vi "DT_With_Multiplexer.vi"() -> (0 "error IO":errorcluster)   [LabVIEW 2017]
doc: "This vi will take data with multiple DT boxes for an arbitrary number of channels either differentially or single ended, depending upon how you have wired the boxes up."
uses:
  Globals/Meas_global.vi
panel:
  in  "DT Board num.":u32=1
  out "Waveform Graph":dbl[][](graph)
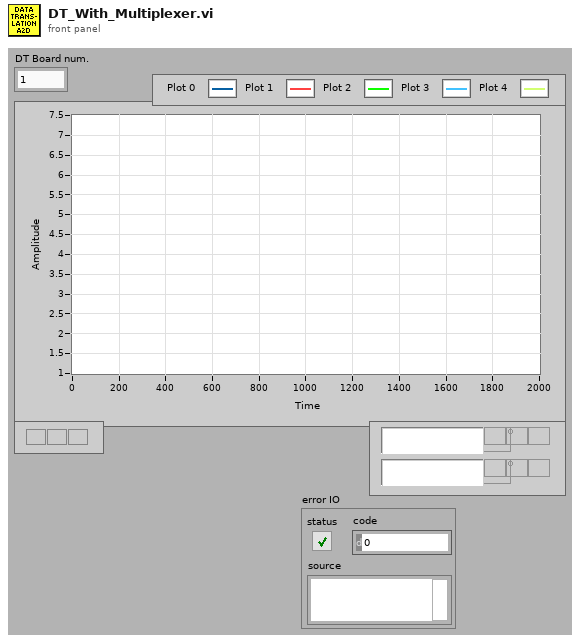
[diagram p1: front panel]
types:
  T1 = typedef "LDA_Setup.ctl" = cluster{"dimensions":enum16{"1D", "2D"}, "Analogue Freq Multiplier":dbl}
  T2 = typedef "Ch_and_Spans.ctl" = cluster{"Sync Delay (ms)":dbl, "Ch No":i16, "Var name":string, "Use Latest Calib":bool}
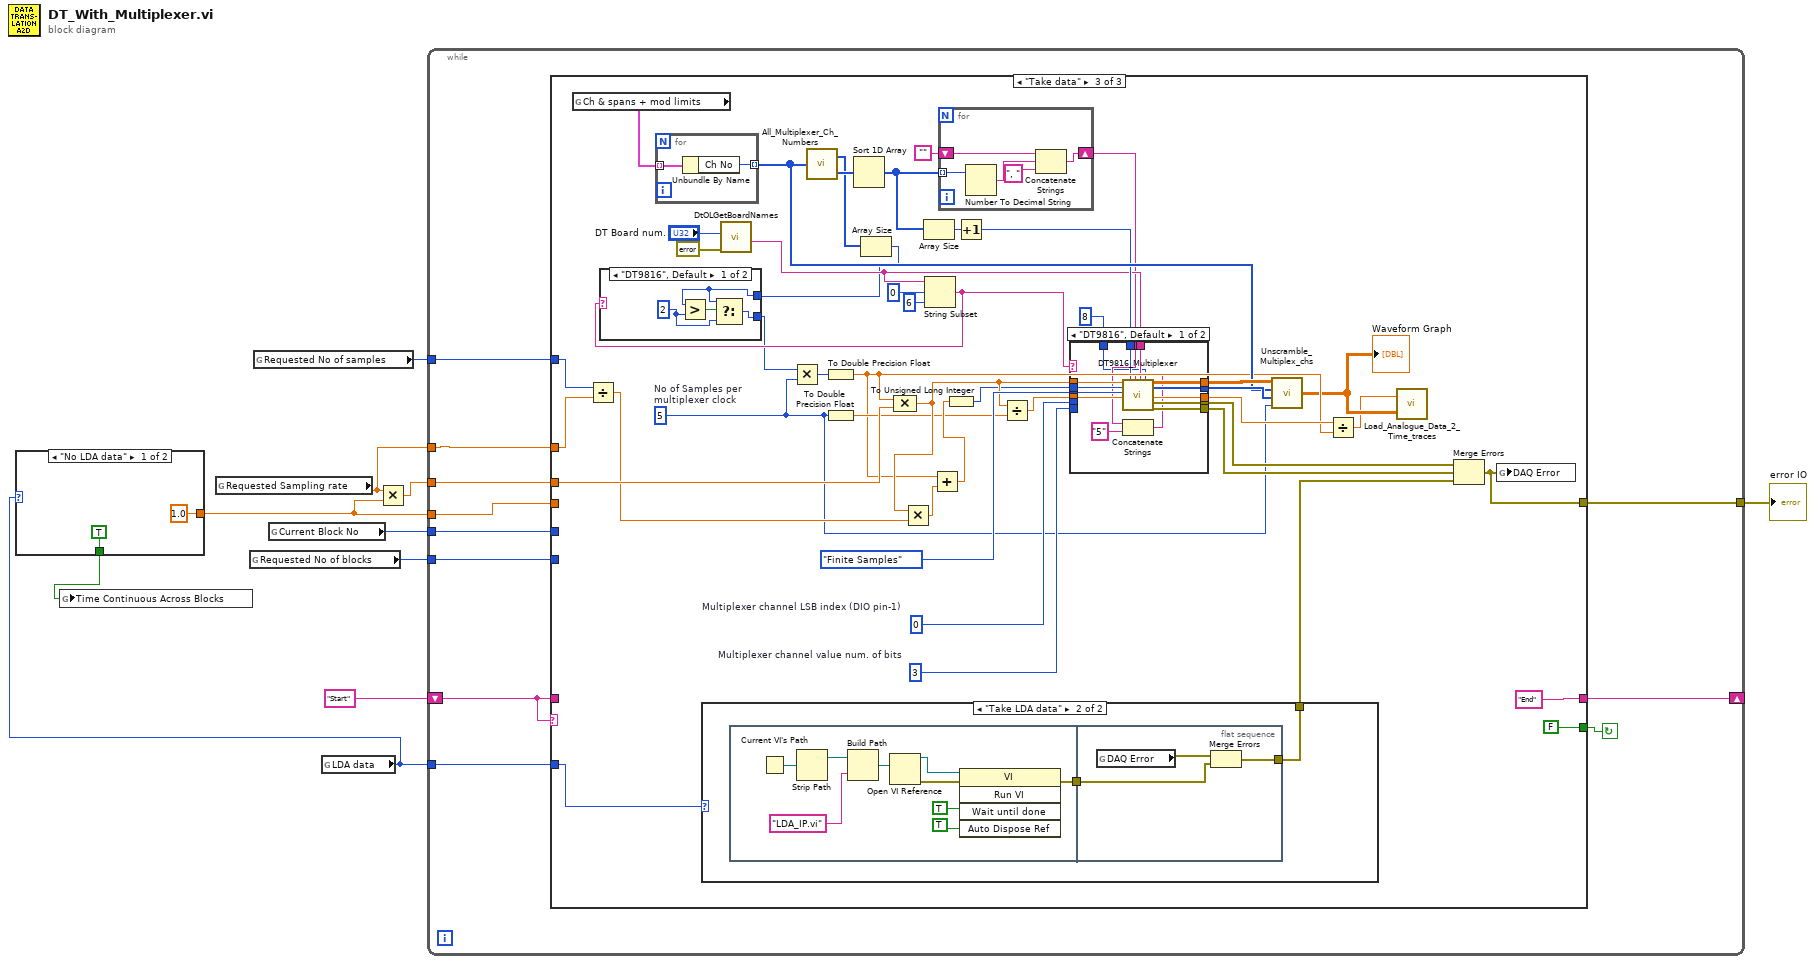
[diagram p0: block diagram]
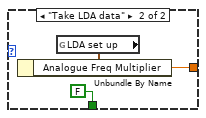
[diagram p2: hidden frame]
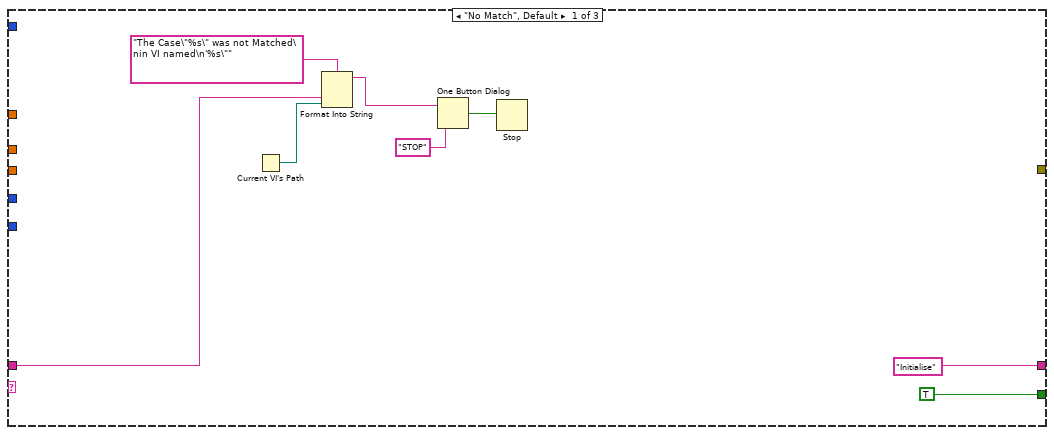
[diagram p3: hidden frame]
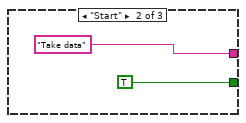
[diagram p4: hidden frame]
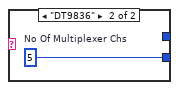
[diagram p5: hidden frame]
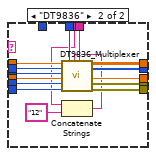
[diagram p6: hidden frame]
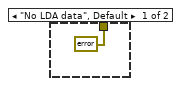
[diagram p7: hidden frame]
diagram:
  n1 = global read "Meas_global.vi" "Requested Sampling rate"() -> (w6:dbl)
  n2 = global read "Meas_global.vi" "Requested No of blocks"() -> (w5:i32)
  n3 = global read "Meas_global.vi" "Requested No of samples"() -> (w9:i32)
  n4 = global read "Meas_global.vi" "Current Block No"() -> (w8:i32)
  n5 = global read "Meas_global.vi" "LDA data"() -> (w3:enum16{"No LDA data", "Take LDA data"})
  n6 = case shown="\"No LDA data\"" w3 {
    tunnel: [1.0 ("Analogue Freq Multiplier") w14] -> w4
    tunnel: [TRUE FALSE] -> w2
    frame "No LDA data" {
    }
    frame "Take LDA data" {
      n7 = global read "Meas_global.vi" "LDA set up"() -> (w15:T1)
      n8 = Unbundle By Name(w15) -> ("Analogue Freq Multiplier"=w14:dbl)
    }
  }
  n9 = global write "Meas_global.vi" "Time Continuous Across Blocks"(w2) -> ()
  n10 = Multiply(x=w6, y=w4) -> (x*y=w7:dbl)
  n11 = while {
    shift-left: "Start" -> [w25]
    shift-right: [w26] -> _
    tunnel: w7 -> [w24]
    tunnel: w9 -> [w23]
    tunnel: w8 -> [w22]
    tunnel: w3 -> [w20]
    tunnel: w4 -> [w19]
    tunnel: w6 -> [w18]
    tunnel: w5 -> [w17]
    tunnel: [w16] -> w1
    stop <- w21 continue-if-true
    n12 = case shown="\"Take data\"" w25 {
      tunnel: ["Initialise" "Take data" "End"] -> w26
      tunnel: w25 -> [w30 _ _]
      tunnel: w24 -> [_ _ w77]
      tunnel: w23 -> [_ _ w76]
      tunnel: w22 -> [_ _ _]
      tunnel: [TRUE TRUE FALSE] -> w21
      tunnel: w20 -> [_ _ w80]
      tunnel: w19 -> [_ _ _]
      tunnel: w18 -> [_ _ w59]
      tunnel: w17 -> [_ _ _]
      tunnel: [_ _ w39] -> w16
      frame "No Match", Default {
        n13 = Current VI's Path() -> (path=w29:path)
        n14 = Format Into String(format string="The Case\"%s\" was not Matched\nin VI named\n'%s\"" ("Format String"), w30, w29) -> (resulting string=w33:string)  [unwired: 2 in, 1 out]
        n15 = One Button Dialog(message=w33, button name ("OK")="STOP") -> (true=w31:bool)
        n16 = Stop(stop? (T)=w31) -> ()
      }
      frame "Start" {
      }
      frame "Take data" {
        w63 = 3  # Multiplexer channel value num. of bits
        w64 = 0  # Multiplexer channel LSB index (DIO pin-1)
        w41 = 5  # No of Samples per multiplexer clock
        n17 = global read "Meas_global.vi" "Ch & spans + mod limits"() -> (w79:T2[])
        n18 = Divide(x=w76, y=w59) -> (x/y=w75:dbl)
        n19 = for {
          tunnel: w79 -> [w125] mode=indexing
          tunnel: [w124] -> w67 mode=indexing
          n20 = Unbundle By Name(w125) -> ("Ch No"=w124:i16)
        }
        n21 = case shown="\"Take LDA data\"" w80 {
          tunnel: [errorcluster {"status"=FALSE, "code"=0, "source"=""} ("error IO") w127] -> w60
          frame "No LDA data", Default {
          }
          frame "Take LDA data" {
            n22 = flat-sequence {
              tunnel: [w129] -> w128
              tunnel: w128 -> [w139]
              tunnel: [w138] -> w127
              frame #0 {
                n23 = Current VI's Path() -> (path=w131:path)
                n24 = Strip Path(path=w131) -> (stripped path=w130:path)  [unwired: 1 out]
                n25 = Build Path(base path=w130, name or relative path="LDA_IP.vi") -> (appended path=w132:path)
                n26 = Open VI Reference(vi path=w132) -> (vi reference=w135:refnum<vi>, error out=w136:errorcluster)  [unwired: 5 in]
                n27 = invoke class="VI" method="Run VI"(reference=w135, error in=w136, "Wait until done"=TRUE ("Wait Until Done"), "Auto Dispose Ref"=TRUE ("Wait until done")) -> (error out=w129:errorcluster)  [unwired: 1 in, 4 out]
              }
              frame #1 {
                n28 = global read "Meas_global.vi" "DAQ Error"() -> (w140:errorcluster)
                n29 = Merge Errors(w140, w139) -> (w138:errorcluster)
              }
            }
          }
        }
        n30 = call <userlib>:"DtOLGetBoardNames.vi"("error in (no error)"=errorcluster {"status"=FALSE, "code"=0, "source"=""}, "Select Board"="DT Board num.") -> ("Board Name"=w49:string)  [unwired: 7 in, 2 out]
        n31 = call "All_Multiplexer_Ch_Numbers.vi"("Channel Numbers"=w67) -> ("Multiplexer Ch No"=w44:i16[], "ADC Ch No"=w58:i16[])
        n32 = To Double Precision Float(number=w41) -> (double precision float=w53:dbl)
        n33 = Sort 1D Array(array=w58) -> (sorted array=w57:i16[])
        n34 = Array Size(array=w44) -> (size(s)=w42:i32)
        n35 = Array Size(array=w57) -> (size(s)=w66:i32)
        n36 = String Subset(string=w49, offset (0)=0, length (rest)=6 ("length (rest)")) -> (substring=w45:string)
        n37 = case shown="\"DT9816\", Default" w45 {
          tunnel: [w83 w87] -> w40
          tunnel: w42 -> [w85 _]
          frame "DT9816", Default {
            w84 = 2 ("y")
            n38 = Greater?(x=w85, y=w84) -> (0:w86:bool)
            n39 = Select(t=w85, s=w86, f=w84) -> (s? t:f=w83:i32)
          }
          frame "DT9836" {
            w87 = 5  # No Of Multiplexer Chs
          }
        }
        n40 = Multiply(x=w40, y=w41) -> (x*y=w52:i32)
        n41 = To Double Precision Float(number=w52) -> (double precision float=w51:dbl)
        n42 = Compound Arithmetic op=MULTIPLY(w51, w77) -> (w71:dbl)
        n43 = Multiply(x=w71, y=w75) -> (x*y=w74:dbl)
        n44 = Add(x=w51, y=w74) -> (x+y=w73:dbl)
        n45 = for {
          tunnel: w57 -> [w123] mode=indexing
          shift-right: [w119] -> w46
          shift-left: "" -> [w120]
          n46 = Number To Decimal String(number=w123) -> (decimal integer string=w122:string)  [unwired: 1 in]
          n47 = Concatenate Strings(w120, w122, ", " ("string")) -> (w119:string)
        }
        n48 = To Unsigned Long Integer(number=w73) -> (unsigned 32bit integer=w50:u32)
        n49 = Increment(x=w66) -> (x+1=w65:i32)
        n50 = Divide(x=w71, y=w53) -> (x/y=w70:dbl)
        n51 = case shown="\"DT9816\", Default" w45 {
          tunnel: w46 -> [w89 w104]
          tunnel: enum16{"Finite Samples", "Continuous Samples"}."Finite Samples" ("Sample Mode") -> [w98 w118]
          tunnel: w71 -> [w100 w117]
          tunnel: w70 -> [w97 w116]
          tunnel: [w93 w115] -> w69
          tunnel: [w92 w114] -> w68
          tunnel: w65 -> [w101 w113]
          tunnel: w64 -> [_ w112]
          tunnel: w63 -> [_ w111]
          tunnel: [w95 w110] -> w62
          tunnel: [w96 w109] -> w61
          tunnel: [w94 w108] -> w56
          tunnel: w49 -> [w102 w107]
          tunnel: w50 -> [w99 w106]
          tunnel: 8 ("size(s)") -> [w88 _]
          frame "DT9816", Default {
            n52 = Concatenate Strings(w89, "5" ("string")) -> (w90:string)
            n53 = call "DT9816_Multiplexer.vi"("Sample Freq (Hz)"=w100, "Samples Per Channel"=w99, "Sample Mode"=w98, "Multiplexer cycle freq. (Hz)"=w97, "Number Chan to Read"=w101, "Channel list (Ain5 for channel volts)"=w90, "Board Name"=w102, "N banks"=w88) -> ("2D volts out"=w92:dbl[][], "Multiplexer bank no."=w93:i32[], "Actual Sample Freq"=w94:dbl, "Data acq. final error"=w95:errorcluster, "Clock error"=w96:errorcluster)  [unwired: 7 in]
          }
          frame "DT9836" {
            n54 = Concatenate Strings(w104, "12" ("string")) -> (w103:string)
            n55 = call "DT9836_Multiplexer.vi"("Sample Freq (Hz)"=w117, "Samples Per Channel"=w106, "Sample Mode"=w118, "Multiplexer cycle freq. (Hz)"=w116, "Multiplexer channel LSB index (DIO pin-1)"=w112, "Multiplexer channel value num. of bits"=w111, "Number Chan to Read"=w113, "Channel list (12 for Digital IO)"=w103, "Board Name"=w107) -> ("2D volts out"=w114:dbl[][], "Multiplexer channel"=w115:u32[], "Actual Sample Freq"=w108:dbl, "Data acq. final error"=w110:errorcluster, "Clock error"=w109:errorcluster)  [unwired: 6 in]
          }
        }
        n56 = call "Unscramble_Multiplex_chs.vi"("No of Samples per multiplexer clock"=w41, "Multiplex Ch No"=w69, "Channel Numbers"=w67, "Voltages"=w68) -> ("Voltage by Req Ch"=w38:dbl[][])
        "Waveform Graph" <- w38
        n57 = Divide(x=w56, y=w51) -> (x/y=w37:dbl)
        n58 = call "Load_Analogue_Data_2_Time_traces.vi"("Voltage Array"=w38, "Sampling Rate (Hz)"=w37) -> ()  [unwired: 1 in]
        n59 = Merge Errors(w62, w61, w60) -> (w39:errorcluster)
        n60 = global write "Meas_global.vi" "DAQ Error"(w39) -> ()
      }
    }
  }
  "error IO" <- w1
